vi "MAT Determine Data Type.vi"(0 "DBL":dbl[][](array[numeric]) format="%.2f", 1 "SGL":sgl[][](array[numeric]) format="%.2f", 2 "I32":i32[][](array[numeric]), 3 "I16":i16[][](array[numeric]), 4 "U16":u16[][](array[numeric]), 5 "U8":u8[][](array[numeric]), 6 "CDB":cdb[][](array[numeric]) format="%.2f", 7 "CSG":csg[][](array[numeric]) format="%.2f", 9 "STR":string[](array[string]), 13 "error in (no error)":errorcluster) -> (10 "Matrix Size":i32[](array[numeric]), 12 "Rep. Code":u32, 14 "Real/Complex (0-Real)":u32, 15 "error out":errorcluster, 17 "Representation":T1, 20 "DBL copy":dbl[][](array[numeric]) format="%.2f", 21 "SGL copy":sgl[][](array[numeric]) format="%.2f", 22 "I32 copy":i32[][](array[numeric]), 23 "I16 copy":i16[][](array[numeric]), 24 "U16 copy":u16[][](array[numeric]), 25 "U8 copy":u8[][](array[numeric]), 26 "CDB copy":cdb[][](array[numeric]) format="%.2f", 27 "CSG copy":csg[][](array[numeric]) format="%.2f")   [LabVIEW 2020]
doc: "A subVI of Save to MAT. If more than one input contains a non-empty array, error is generated (error code 501)."
uses:
  MAT Type Representation.ctl
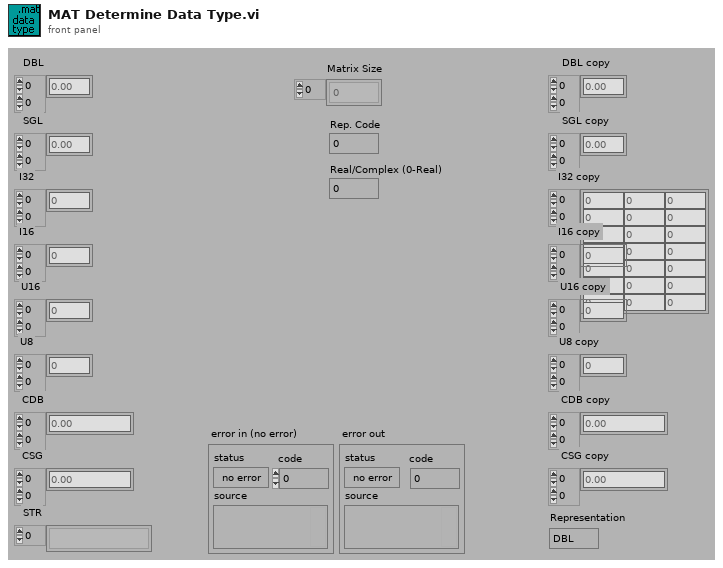
[diagram p1: front panel]
types:
  T1 = typedef "MAT Type Representation.ctl" = enum16{"DBL", "SGL", "I32", "I16", "U16", "U8", "CDB", "CSG", "STR"}
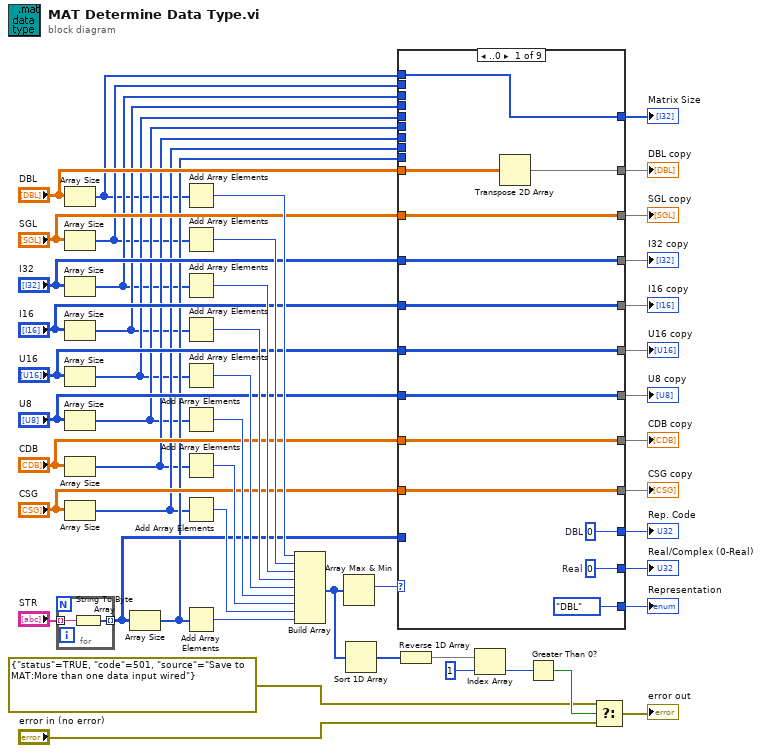
[diagram p0: block diagram]
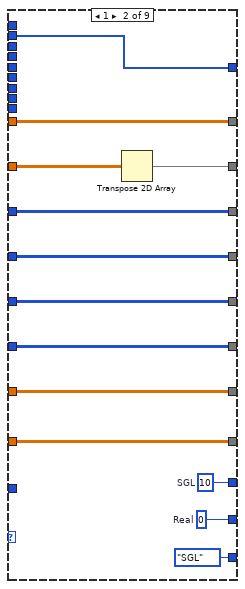
[diagram p2: hidden frame]
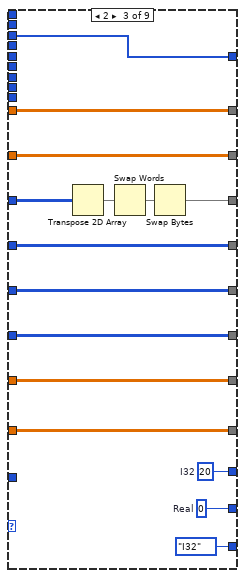
[diagram p3: hidden frame]
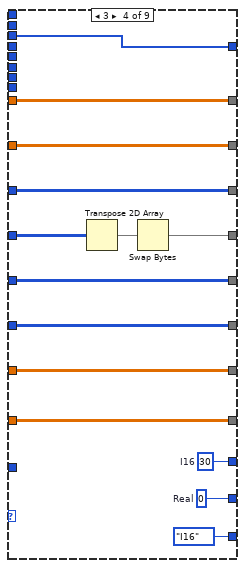
[diagram p4: hidden frame]
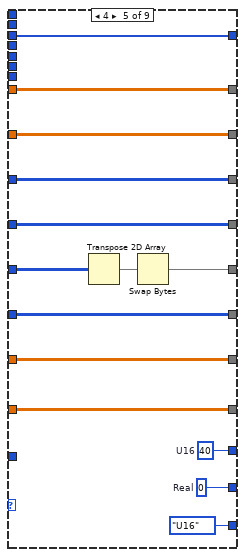
[diagram p5: hidden frame]
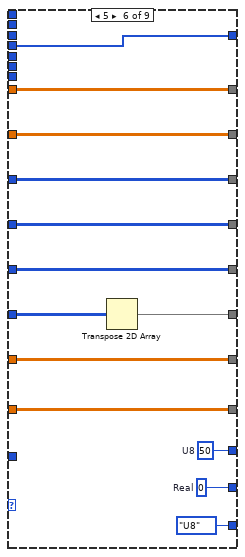
[diagram p6: hidden frame]
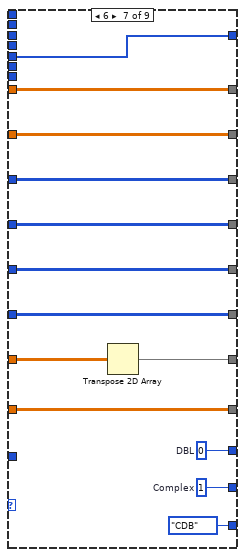
[diagram p7: hidden frame]
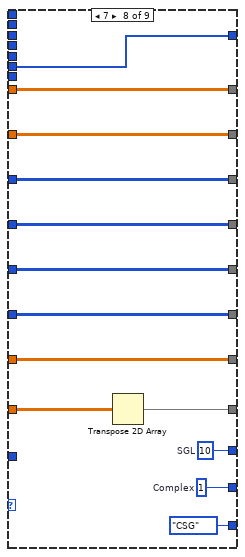
[diagram p8: hidden frame]
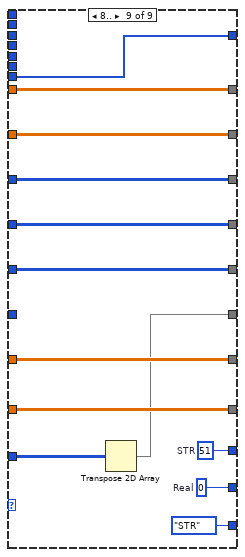
[diagram p9: hidden frame]
diagram:
  n1 = for {
    tunnel: "STR" -> [w52] mode=indexing
    tunnel: [w51] -> w24 mode=indexing
    n2 = String To Byte Array(string=w52) -> (unsigned byte array=w51:u8[])
  }
  n3 = Array Size(array="DBL") -> (size(s)=w13:i32[])
  n4 = Array Size(array="SGL") -> (size(s)=w14:i32[])
  n5 = Array Size(array="I32") -> (size(s)=w15:i32[])
  n6 = Array Size(array="I16") -> (size(s)=w16:i32[])
  n7 = Array Size(array="U16") -> (size(s)=w17:i32[])
  n8 = Array Size(array="U8") -> (size(s)=w18:i32[])
  n9 = Array Size(array="CDB") -> (size(s)=w19:i32[])
  n10 = Array Size(array="CSG") -> (size(s)=w20:i32[])
  n11 = Array Size(array=w24) -> (size(s)=w21:i32[])
  n12 = Add Array Elements(numeric array=w13) -> (sum=w49:i32)
  n13 = Add Array Elements(numeric array=w14) -> (sum=w48:i32)
  n14 = Add Array Elements(numeric array=w15) -> (sum=w47:i32)
  n15 = Add Array Elements(numeric array=w16) -> (sum=w46:i32)
  n16 = Add Array Elements(numeric array=w17) -> (sum=w45:i32)
  n17 = Add Array Elements(numeric array=w18) -> (sum=w44:i32)
  n18 = Add Array Elements(numeric array=w19) -> (sum=w43:i32)
  n19 = Add Array Elements(numeric array=w20) -> (sum=w42:i32)
  n20 = Add Array Elements(numeric array=w21) -> (sum=w41:i32)
  n21 = Build Array(w49, w48, w47, w46, w45, w44, w43, w42, w41) -> (w9:i32[])
  n22 = Array Max & Min(array=w9) -> (max index (indices)=w11:i32)  [unwired: 3 out]
  n23 = Sort 1D Array(array=w9) -> (sorted array=w7:i32[])
  n24 = case shown="..0" w11 {
    tunnel: [w65 w78 w93 w107 w121 w134 w147 w160 w173] -> w23
    tunnel: [w64 w77 w92 w106 w120 w133 w146 w159 w172] -> w22
    tunnel: "DBL" -> [w55 w70 w86 w101 w116 w130 w144 w158 w171]
    tunnel: "SGL" -> [w63 w68 w85 w100 w115 w129 w143 w157 w170]
    tunnel: "I32" -> [w62 w76 w81 w99 w114 w128 w142 w156 w169]
    tunnel: "I16" -> [w61 w75 w91 w96 w112 w127 w141 w155 w168]
    tunnel: "U16" -> [w60 w74 w90 w105 w110 w126 w140 w154 w167]
    tunnel: "U8" -> [w59 w73 w89 w104 w119 w124 w139 w153 _]
    tunnel: "CDB" -> [w58 w72 w88 w103 w118 w132 w137 w152 w166]
    tunnel: "CSG" -> [w57 w71 w87 w102 w117 w131 w145 w150 w165]
    tunnel: [w56 w70 w86 w101 w116 w130 w144 w158 w171] -> w31
    tunnel: [w63 w69 w85 w100 w115 w129 w143 w157 w170] -> w30
    tunnel: [w62 w76 w82 w99 w114 w128 w142 w156 w169] -> w29
    tunnel: [w61 w75 w91 w97 w112 w127 w141 w155 w168] -> w28
    tunnel: [w59 w73 w89 w104 w119 w125 w139 w153 w164] -> w26
    tunnel: [w57 w71 w87 w102 w117 w131 w145 w151 w165] -> w32
    tunnel: [w60 w74 w90 w105 w111 w126 w140 w154 w167] -> w27
    tunnel: [w58 w72 w88 w103 w118 w132 w138 w152 w166] -> w25
    tunnel: w24 -> [_ _ _ _ _ _ _ _ w163]
    tunnel: w21 -> [_ _ _ _ _ _ _ _ w162]
    tunnel: w20 -> [_ _ _ _ _ _ _ w149 _]
    tunnel: w19 -> [_ _ _ _ _ _ w136 _ _]
    tunnel: w18 -> [_ _ _ _ _ w123 _ _ _]
    tunnel: w17 -> [_ _ _ _ w109 _ _ _ _]
    tunnel: w16 -> [_ _ _ w95 _ _ _ _ _]
    tunnel: w15 -> [_ _ w80 _ _ _ _ _ _]
    tunnel: w14 -> [_ w67 _ _ _ _ _ _ _]
    tunnel: w13 -> [w54 _ _ _ _ _ _ _ _]
    tunnel: [w54 w67 w80 w95 w109 w123 w136 w149 w162] -> w12
    tunnel: [MAT_Type_Representation."DBL" ("Representation") MAT_Type_Representation."SGL" ("Representation") MAT_Type_Representation."I32" ("Representation") MAT_Type_Representation."I16" ("Representation") MAT_Type_Representation."U16" ("Representation") MAT_Type_Representation."U8" ("Representation") MAT_Type_Representation."CDB" ("Representation") MAT_Type_Representation."CSG" ("Representation") MAT_Type_Representation."STR" ("Representation")] -> w10
    frame ..0 {
      w64 = u32 0  # Real
      w65 = u32 0  # DBL
      n25 = Transpose 2D Array(2D array=w55) -> (transposed array=w56:dbl[][])
    }
    frame 1 {
      w77 = u32 0  # Real
      w78 = u32 10  # SGL
      n26 = Transpose 2D Array(2D array=w68) -> (transposed array=w69:sgl[][])
    }
    frame 2 {
      w92 = u32 0  # Real
      w93 = u32 20  # I32
      n27 = Transpose 2D Array(2D array=w81) -> (transposed array=w84:i32[][])
      n28 = Swap Words(1:w84) -> (0:w83:i32[][])
      n29 = Swap Bytes(anything=w83) -> (byte swapped=w82:i32[][])
    }
    frame 3 {
      w106 = u32 0  # Real
      w107 = u32 30  # I16
      n30 = Transpose 2D Array(2D array=w96) -> (transposed array=w98:i16[][])
      n31 = Swap Bytes(anything=w98) -> (byte swapped=w97:i16[][])
    }
    frame 4 {
      w120 = u32 0  # Real
      w121 = u32 40  # U16
      n32 = Transpose 2D Array(2D array=w110) -> (transposed array=w113:u16[][])
      n33 = Swap Bytes(anything=w113) -> (byte swapped=w111:u16[][])
    }
    frame 5 {
      w133 = u32 0  # Real
      w134 = u32 50  # U8
      n34 = Transpose 2D Array(2D array=w124) -> (transposed array=w125:u8[][])
    }
    frame 6 {
      w146 = u32 1  # Complex
      w147 = u32 0  # DBL
      n35 = Transpose 2D Array(2D array=w137) -> (transposed array=w138:cdb[][])
    }
    frame 7 {
      w159 = u32 1  # Complex
      w160 = u32 10  # SGL
      n36 = Transpose 2D Array(2D array=w150) -> (transposed array=w151:csg[][])
    }
    frame 8.. {
      w172 = u32 0  # Real
      w173 = u32 51  # STR
      n37 = Transpose 2D Array(2D array=w163) -> (transposed array=w164:u8[][])
    }
  }
  "DBL copy" <- w31
  "SGL copy" <- w30
  "CSG copy" <- w32
  "I32 copy" <- w29
  "I16 copy" <- w28
  "U16 copy" <- w27
  "U8 copy" <- w26
  "CDB copy" <- w25
  "Matrix Size" <- w12
  "Rep. Code" <- w23
  "Real/Complex (0-Real)" <- w22
  "Representation" <- w10
  n38 = Reverse 1D Array(array=w7) -> (reversed array=w6:i32[])
  n39 = Index Array(array=w6, index=1) -> (element=w5:i32)
  n40 = Greater Than 0?(x=w5) -> (x > 0?=w4:bool)
  n41 = Select(t=errorcluster {"status"=TRUE, "code"=501, "source"="Save to MAT:More than one data input wired"} ("error in (no error)"), s=w4, f="error in (no error)") -> (s? t:f=→"error out":errorcluster)
